vi "Close.vi"(8 "error in (no error)":errorcluster, 11 "KE65XX DMM in":refnum<class "Keithley 65XX DMM.lvclass">) -> (0 "error out":errorcluster, 3 "KE65XX DMM out":refnum<class "Keithley 65XX DMM.lvclass">)   [LabVIEW 2025, in "DMM.lvlib" / "Keithley 65XX DMM.lvclass"]
uses:
  Keithley 65XX DMM.lvclass
  Keithley 65XX DMM.lvclass/Keithley 65XX DMM.ctl
  <instrlib>/Keithley DMM6500 DAQ6500 Series/Keithley DMM6500 DAQ6500 Series.lvlib
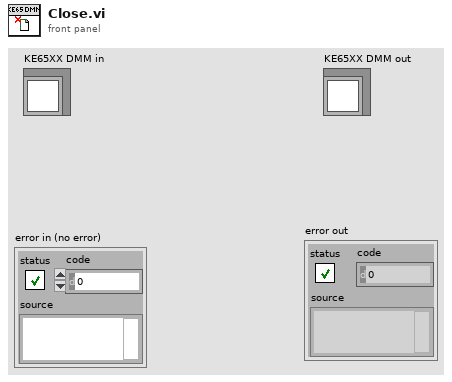
[diagram p1: front panel]
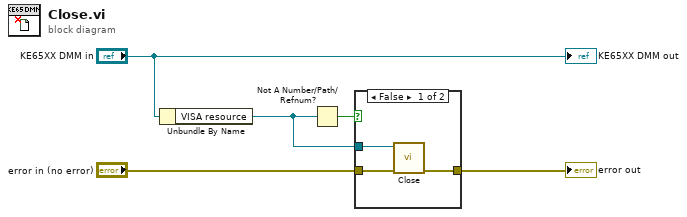
[diagram p0: block diagram]
diagram:
  n1 = Unbundle By Name("KE65XX DMM in") -> ("VISA resource"=w3:refnum<visa-resource-name>)
  n2 = Not A Number/Path/Refnum?(number/path/refnum=w3) -> (NaN/Path/Refnum?=w4:bool)
  n3 = case shown="False" w4 {
    tunnel: "error in (no error)" -> [w7 w9]
    tunnel: [w6 w9] -> w1
    tunnel: w3 -> [w8 _]
    frame False {
      n4 = call <instrlib>:"Close.vi"("error in (no error)"=w7, "VISA resource name"=w8) -> ("error out"=w6:errorcluster)  [unwired: 9 in]
    }
    frame True {
    }
  }
  "error out" <- w1
  "KE65XX DMM out" <- "KE65XX DMM in"
